vi "Config Binding.vi"(8 "error in (no error)":errorcluster, 11 "Configuration in":refnum<class "Configuration.lvclass">) -> (0 "error out":errorcluster, 3 "Configuration out":refnum<class "Configuration.lvclass">)   [LabVIEW 2016, in "Hardware.lvlib" / "Motions.lvlib" / "Motions Configuration.lvclass"]
uses:
  <userlib>/Common Components/Hardware/Abstract System/Motions/Motions Config/Motions Configuration.lvclass
  <userlib>/Configuration Dialog Actor/Configuration.lvclass
  C:/Program Files (x86)/National Instruments/LabVIEW 2016/user.lib/Configuration Dialog Actor/Configuration.lvclass
  C:/Program Files (x86)/National Instruments/LabVIEW 2016/vi.lib/ActorFramework/Actor/Actor.lvclass
  <userlib>/Common Components/Hardware/Abstract System/Motions/Motions Config/Motions Configuration.lvclass/Motions Configuration.ctl
  <vilib>/ActorFramework/Actor/Actor.lvclass/Actor.ctl
  <userlib>/Common Components/Hardware/Abstract System/Motions/Motions/Motions.lvclass/Motions.ctl
  <userlib>/Common Components/Hardware/Abstract System/Motions/Motions/Motions.lvclass
  <vilib>/ActorFramework/Actor/Actor.lvclass
panel:
  in  "TA Binding List":i32(listbox)
  in  "Revert":bool
  # "back to the state when you entered this page."
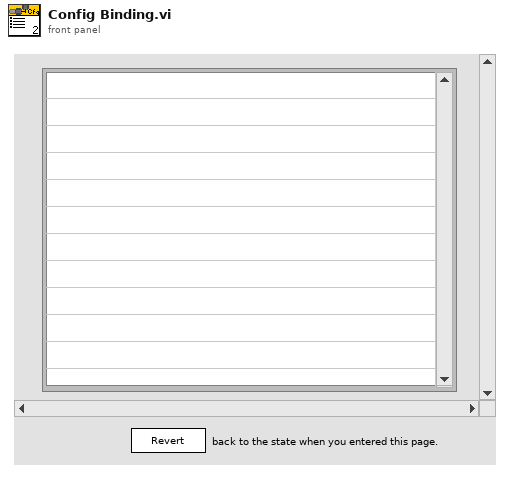
[diagram p1: front panel]
types:
  T1 = typedef "Hardware.lvlib/Motions.lvlib/Motions.lvclass/TA Binding Data.ctl" = cluster{"Triggers":cluster{"Triggers for Array AND":cluster{"Index":u8, "State Name":string}[]}[], "Actions":cluster{"Action Name":string, "Action Data":string}[]}
  T2 = typedef "eventvkey.ctl" = enum16{"ASCII", "Enter", "Return", "Shift", "Ctrl", "Alt", "Cmd", "Opt", "Caps", "NumLock", "Clear", "Break", "Up", "Down", "Left", "Right", "Insert", "Delete", "Home", "End", "PageUp", "PageDown", "Escape", "Help", "Pause", "ScrollLock", "F1", "F2", "F3", "F4", "F5", "F6", "F7", "F8", "F9", "F10", "F11", "F12", "F13", "F14", "F15", "F16", "F17", "F18", "F19", "F20", "F21", "F22", "F23", "F24", "Play", "VolumeUp", "VolumeDown", "Mute", "Two Byte Char"}
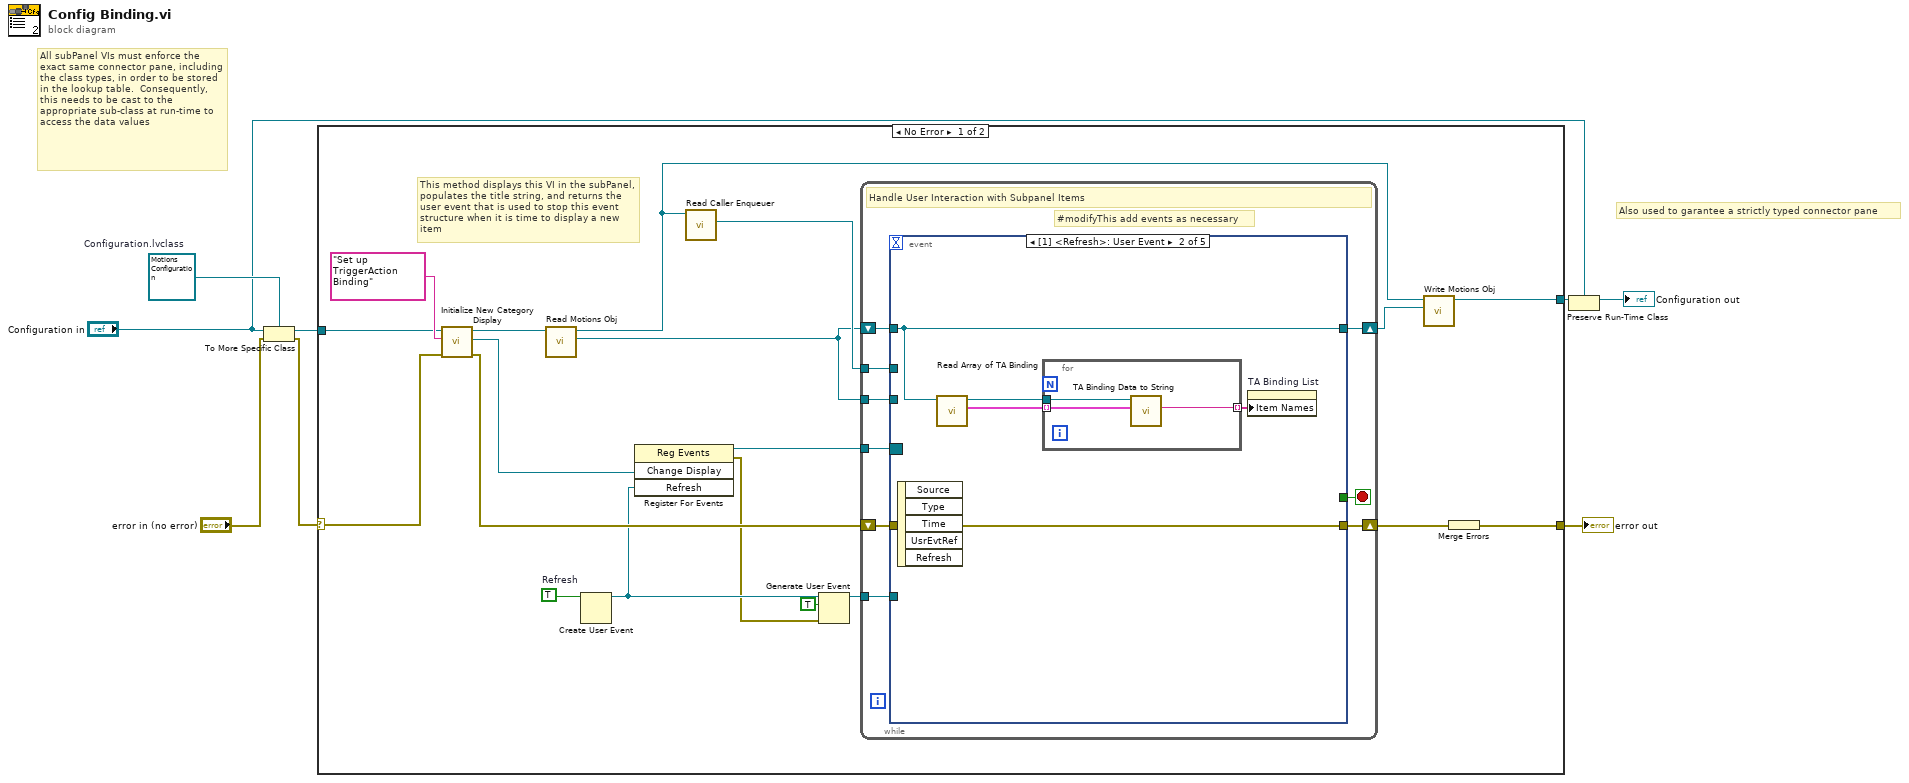
[diagram p0: block diagram]
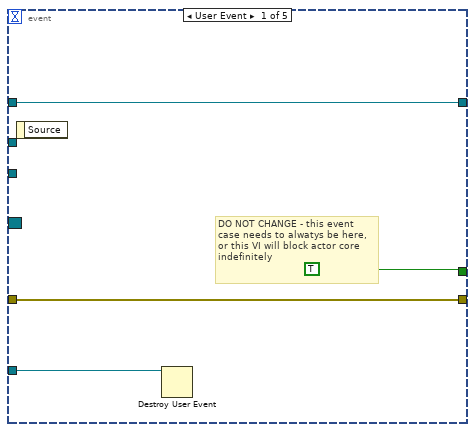
[diagram p2: hidden frame]
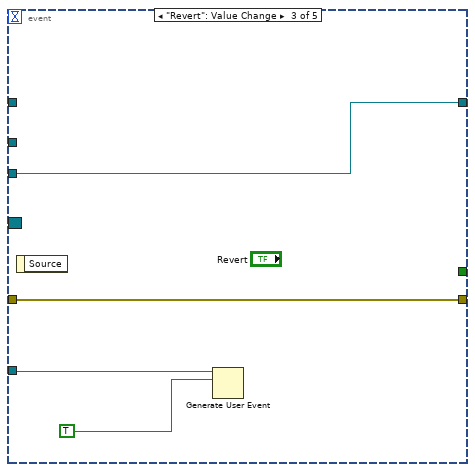
[diagram p3: hidden frame]
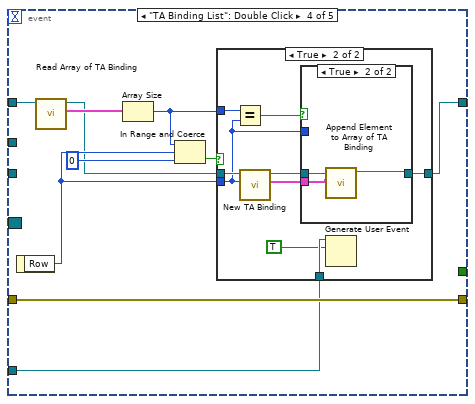
[diagram p4: hidden frame]
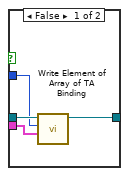
[diagram p6: hidden frame]
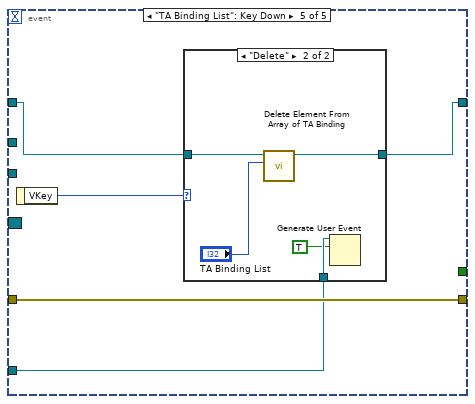
[diagram p7: hidden frame]
diagram:
  w5 = refnum<class "Motions Configuration.lvclass"> refnum  # Configuration.lvclass
  # "Also used to garantee a strictly typed connector pane"
  # "All subPanel VIs must enforce the exact same connector pane, including the class types, in order to be stored in the lookup table.  Consequently, this needs to be cast to the appropriate sub-class at run-time to access the data values"
  n1 = To More Specific Class(target class=w5, reference="Configuration in", error in="error in (no error)") -> (specific class reference=w6:refnum<class "Motions Configuration.lvclass">, error out=w1:errorcluster)
  n2 = case shown="No Error" w1 {
    selector: w1 -> [w26 w91]
    tunnel: w6 -> [w19 w92]
    tunnel: [w13 w92] -> w8
    tunnel: [w27 w91] -> w7
    frame No Error {
      w18 = TRUE  # Refresh
      # "This method displays this VI in the subPanel, populates the title string, and returns the user event that is used to stop this event structure when it is time to display a new item"
      n3 = call <userlib>:"Initialize New Category Display.vi"("error in (no error)"=w26, "Name to Display"="Set up TriggerAction Binding", "Configuration in"=w19) -> ("error out"=w21:errorcluster, "Change Display"=w24:refnum<user-event>, "Configuration Out"=w15:refnum<class "Motions Configuration.lvclass">)  [unwired: 6 in]
      n4 = call <userlib>:"Read Motions Obj.vi"("Motions Configuration in"=w15) -> ("Hardware.lvlib:Motions.lvlib:Motions.lvclass"=w16:refnum<class "Motions.lvclass">, "Motions Configuration out"=w14:refnum<class "Motions Configuration.lvclass">)  [unwired: 8 in, 1 out]
      n5 = Create User Event(user event datatype=w18) -> (user event=w17:refnum<user-event>)  [unwired: 1 in, 1 out]
      n6 = register-events(w24, w17) -> (reference out=w23:refnum<event-registration>, error out=w9:errorcluster)  [unwired: 2 in]
      n7 = call <vilib>:"Read Caller Enqueuer.vi"("Actor"=w14) -> ("Caller Enqueuer"=w20:refnum<class "Message Enqueuer.lvclass">)  [unwired: 10 in]
      n8 = Generate User Event(user event=w17, event data cluster=TRUE ("event data"), error in=w9) -> (user event out=w11:refnum<user-event>)  [unwired: 1 in, 1 out]
      n9 = while {
        tunnel: w23 -> [w35]
        shift-right: [w34] -> w22
        shift-left: w21 -> [w33]
        tunnel: w20 -> [w32]
        tunnel: w16 -> [w31]
        tunnel: w11 -> [w30]
        shift-right: [w28] -> w12
        shift-left: w16 -> [w29]
        stop <- w36 stop-if-true
        # "#modifyThis add events as necessary"
        # "Handle User Interaction with Subpanel Items"
        n10 = event shown="[1] <Refresh>: User Event" {
          selector: w35 -> [_ _ _ _ _]
          dyn-events: _ -> [_ _ _ _ _]
          timeout: _ -> [_ _ _ _ _]
          tunnel: [TRUE _ _ _ _] -> w36
          tunnel: [w40 w45 w52 w62 w84] -> w34
          tunnel: w33 -> [w40 w45 w52 w62 w84]
          tunnel: w32 -> [_ _ _ _ _]
          tunnel: w31 -> [_ _ w49 _ _]
          tunnel: w30 -> [w38 _ w51 w57 w82]
          tunnel: w29 -> [w37 w43 _ w55 w81]
          tunnel: [w37 w43 w49 w54 w80] -> w28
          event User Event {
            # "DO NOT CHANGE - this event case needs to alwatys be here, or this VI will block actor core indefinitely"
            n11 = event-data() -> ()  [unwired: 1 in, 1 out]
            n12 = Destroy User Event(user event=w38) -> ()  [unwired: 1 in, 1 out]
          }
          event User Event {
            n13 = event-data() -> ()  [unwired: 1 in, 5 out]
            n14 = call <userlib>:"Read Array of TA Binding.vi"("Motions in"=w43) -> ("Array of TA Binding"=w41:T1[], "Motions out"=w42:refnum<class "Motions.lvclass">)  [unwired: 9 in]
            n15 = for {
              tunnel: w41 -> [w48] mode=indexing
              tunnel: [w47] -> w44 mode=indexing
              tunnel: w42 -> [w46]
              n16 = call <userlib>:"TA Binding Data to String.vi"("TA Binding Data"=w48, "Motions in"=w46) -> ("String"=w47:string)  [unwired: 7 in, 2 out]
            }
            n17 = property on="TA Binding List" class="LstBox (strict)"("Item Names"=w44) -> ()  [unwired: 2 in, 2 out]
          }
          event "Revert": Value Change {
            n18 = event-data() -> ()  [unwired: 1 in, 1 out]
            n19 = Generate User Event(user event=w51, event data cluster=TRUE) -> ()  [unwired: 2 in, 2 out]
          }
          event "TA Binding List": Double Click {
            n20 = event-data() -> ("Row"=w61:i32)  [unwired: 1 in]
            n21 = call <userlib>:"Read Array of TA Binding.vi"("Motions in"=w55) -> ("Array of TA Binding"=w56:T1[], "Motions out"=w53:refnum<class "Motions.lvclass">)  [unwired: 9 in]
            n22 = Array Size(array=w56) -> (size(s)=w58:i32)
            n23 = In Range and Coerce(upper limit=w58, x=w61, lower limit=0) -> (In Range?=w59:bool)  [unwired: 1 out]
            n24 = case shown="True" w59 {
              tunnel: w53 -> [w63 w72]
              tunnel: w61 -> [_ w68]
              tunnel: w58 -> [_ w71]
              tunnel: w57 -> [_ w67]
              tunnel: [w63 w64] -> w54
              frame False {
              }
              frame True {
                n25 = Equal?(x=w71, y=w68) -> (x = y?=w70:bool)
                n26 = call <userlib>:"New TA Binding.vi"("Index (out of array range means creating new)"=w68, "Motions in"=w72) -> ("New TA Binding out"=w69:T1, "Motions out"=w65:refnum<class "Motions.lvclass">)  [unwired: 7 in, 1 out]
                n27 = case shown="True" w70 {
                  tunnel: w69 -> [w75 w78]
                  tunnel: w68 -> [w74 _]
                  tunnel: w65 -> [w76 w79]
                  tunnel: [w73 w77] -> w64
                  frame False {
                    n28 = call <userlib>:"Write Element of Array of TA Binding.vi"("Cluster"=w75, "index"=w74, "Motions in"=w76) -> ("Motions out"=w73:refnum<class "Motions.lvclass">)  [unwired: 8 in]
                  }
                  frame True {
                    n29 = call <userlib>:"Append Element to Array of TA Binding.vi"("Cluster"=w78, "Motions in"=w79) -> ("Motions out"=w77:refnum<class "Motions.lvclass">)  [unwired: 9 in]
                  }
                }
                n30 = Generate User Event(user event=w67, event data cluster=TRUE) -> ()  [unwired: 2 in, 2 out]
              }
            }
          }
          event "TA Binding List": Key Down {
            n31 = event-data() -> ("VKey"=w83:T2)  [unwired: 1 in]
            n32 = case shown="\"Delete\"" w83 {
              tunnel: w82 -> [_ w90]
              tunnel: w81 -> [w85 w88]
              tunnel: [w85 w87] -> w80
              frame Default {
              }
              frame "Delete" {
                n33 = call <userlib>:"Delete Element From Array of TA Binding.vi"("index"="TA Binding List", "Motions in"=w88) -> ("Motions out"=w87:refnum<class "Motions.lvclass">)  [unwired: 9 in]
                n34 = Generate User Event(user event=w90, event data cluster=TRUE) -> ()  [unwired: 2 in, 2 out]
              }
            }
          }
        }
      }
      n35 = call <userlib>:"Write Motions Obj.vi"("Hardware.lvlib:Motions.lvlib:Motions.lvclass"=w12, "Motions Configuration in"=w14) -> ("Motions Configuration out"=w13:refnum<class "Motions Configuration.lvclass">)  [unwired: 8 in, 1 out]
      n36 = Merge Errors(w22) -> (w27:errorcluster)
    }
    frame Error {
    }
  }
  "error out" <- w7
  n37 = Preserve Run-Time Class(object in=w8, 2:"Configuration in") -> (object out=→"Configuration out":refnum<class "Configuration.lvclass">)  [unwired: 1 in, 1 out]
